vi "Get niRfsaBT Handles.vi"(8 "error in (no error)":errorcluster, 11 "niDTS BT Tx Test in":refnum<class "niDTS BT Tx Test.lvclass">) -> (0 "error out":errorcluster, 2 "niRfsaBT Handles":T1[][](array[typedef]), 3 "niDTS BT Tx Test out":refnum<class "niDTS BT Tx Test.lvclass">)   [LabVIEW 2015, in "niDTS BT.lvlib" / "niDTS BT Tx Test.lvclass"]
uses:
  niDTS BT Tx Test.lvclass
  RiviInstDriver/niRfsaBT/Includes/niRfsaBt INC Handle.ctl
  RiviInstDriver/niRfsaBT/Objects/niRfsaBt.lvclass
  niDTS BT Tx Test.lvclass/niDTS BT Tx Test.ctl
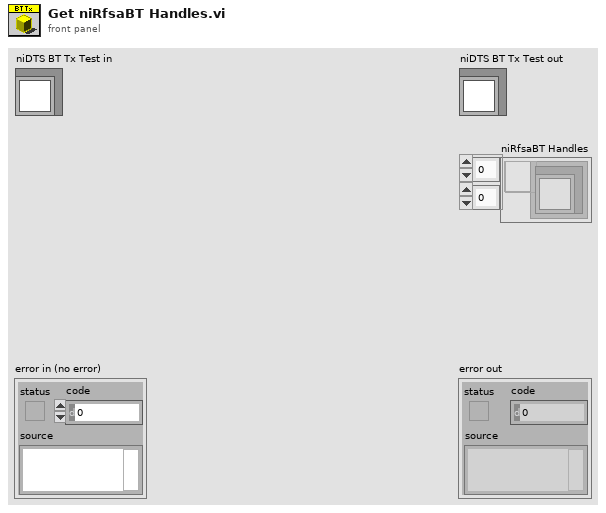
[diagram p1: front panel]
types:
  T1 = typedef "niRfsaBT.lvclass/niRfsaBT INC Handle.ctl" = refnum<data-value>
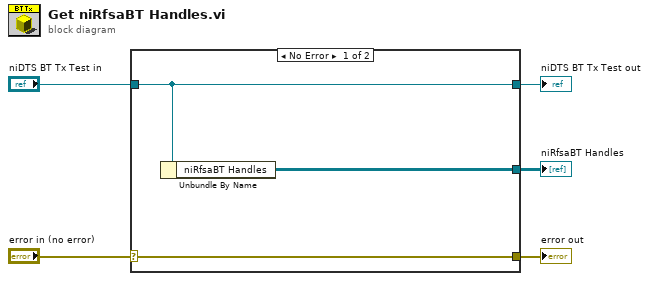
[diagram p0: block diagram]
diagram:
  n1 = case shown="No Error" "error in (no error)" {
    selector: "error in (no error)" -> [w8 w9]
    tunnel: [w8 w9] -> w4
    tunnel: [w7 w10] -> w2
    tunnel: "niDTS BT Tx Test in" -> [w7 w10]
    tunnel: [w6 _] -> w1
    frame No Error {
      n2 = Unbundle By Name(w7) -> ("niRfsaBT Handles"=w6:T1[][])
    }
    frame Error {
    }
  }
  "error out" <- w4
  "niDTS BT Tx Test out" <- w2
  "niRfsaBT Handles" <- w1
